vi "createConnection.vi"(8 "error in (no error)":errorcluster, 11 "ModernOvenFactory In":refnum<class "ModernOvenFactory.lvclass">) -> (0 "error out":errorcluster, 2 "connection":refnum<class "IConnection.lvclass">, 3 "ModernOvenFactory Out":refnum<class "ModernOvenFactory.lvclass">)   [LabVIEW 2023, in "AbstractFactory.lvlib" / "ModernOvenFactory.lvclass"]
uses:
  ModernOvenFactory.lvclass
  IConnection/IConnection.lvclass
  ModernOvenFactory.lvclass/ModernOvenFactory.ctl
  TCPConnection/TCPConnection.lvclass
  C:/projects/DesignPatterns_LabVIEW/AbstractFactory/TCPConnection/TCPConnection.lvclass
  C:/projects/DesignPatterns_LabVIEW/AbstractFactory/IConnection/IConnection.lvclass
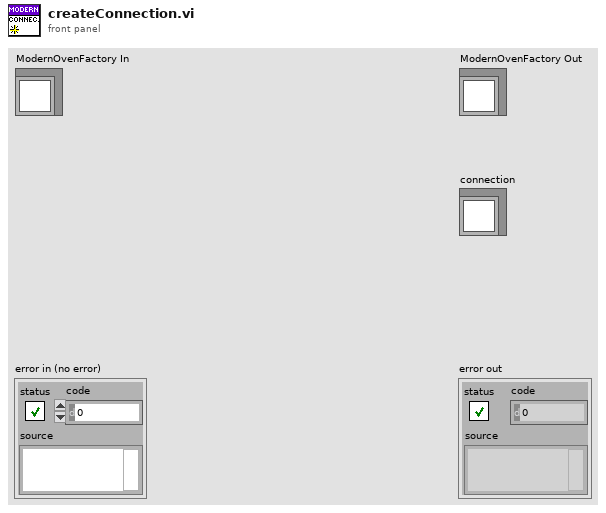
[diagram p1: front panel]
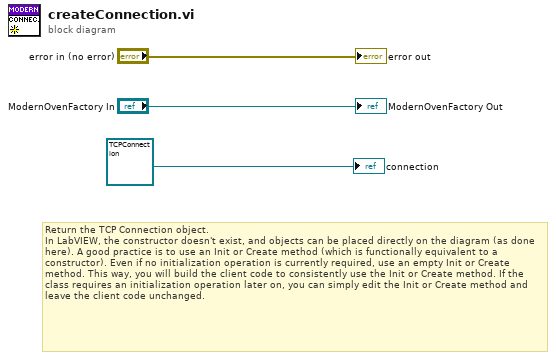
[diagram p0: block diagram]
diagram:
  # "Return the TCP Connection object.\nIn LabVIEW, the constructor doesn't exist, and objects can be placed directly on the diagram (as done here). A good practice is to use an Init or Create method (which is functionally equivalent to a constructor). Even if no initialization operation is currently required, use an empty Init or Create method. This way, you will build the client code to consistently use the Init or Create method. If the class requires an initialization operation later on, you can simply edit the Init or Create method and leave the client code unchanged."
  "error out" <- "error in (no error)"
  "ModernOvenFactory Out" <- "ModernOvenFactory In"
  "connection" <- refnum<class "TCPConnection.lvclass"> refnum ("AbstractFactory.lvlib:TCPConnection.lvclass")
